vi "Happen YAML.vi"(4 "Condensed?":bool=TRUE, 6 "No Label?":bool, 8 "error in (no error)":errorcluster, 9 "Level":u32, 10 "Anything":variant, 11 "YAML String in":string) -> (0 "error out":errorcluster, 3 "YAML String out":string)   [LabVIEW 2015, in "YAML Parser.lvlib"]
uses:
  YAML Parser.lvlib
  <vilib>/Utility/Data Type/Type Definitions/Data Type.ctl
  <vilib>/Utility/Data Type/NI_Data Type.lvlib
  <vilib>/Utility/error.llb/whitespace.ctl
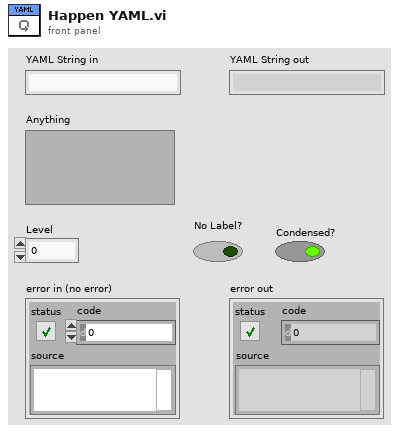
[diagram p1: front panel]
types:
  T1 = typedef "NI_Data Type.lvlib/Data Type.ctl" = enum8{"Invalid Type", "Void", "I8", "I16", "I32", "I64", "U8", "U16", "U32", "U64", "Single Float", "Double Float", "Extended Float", "Single Complex", "Double Complex", "Extended Complex", "Enum U8", "Enum U16", "Enum U32", "Enum U64", "Single Float With Unit", "Double Float With Unit", "Extended Float With Unit", "Single Complex with Unit", "Double Complex with Unit", "Extended Complex with Unit", "Boolean", "String", "Path", "Picture", "Tag", "Array", "Cluster", "Variant", "LV Variant", "Waveform", "Timestamp", "Digital Waveform", "Digital Data", "ExpressData", "Refnum", "External Data", "VI", "Poly VI", "LabVIEW Class Instance", "Fixed Point"}
  T2 = typedef "whitespace.ctl" = u16
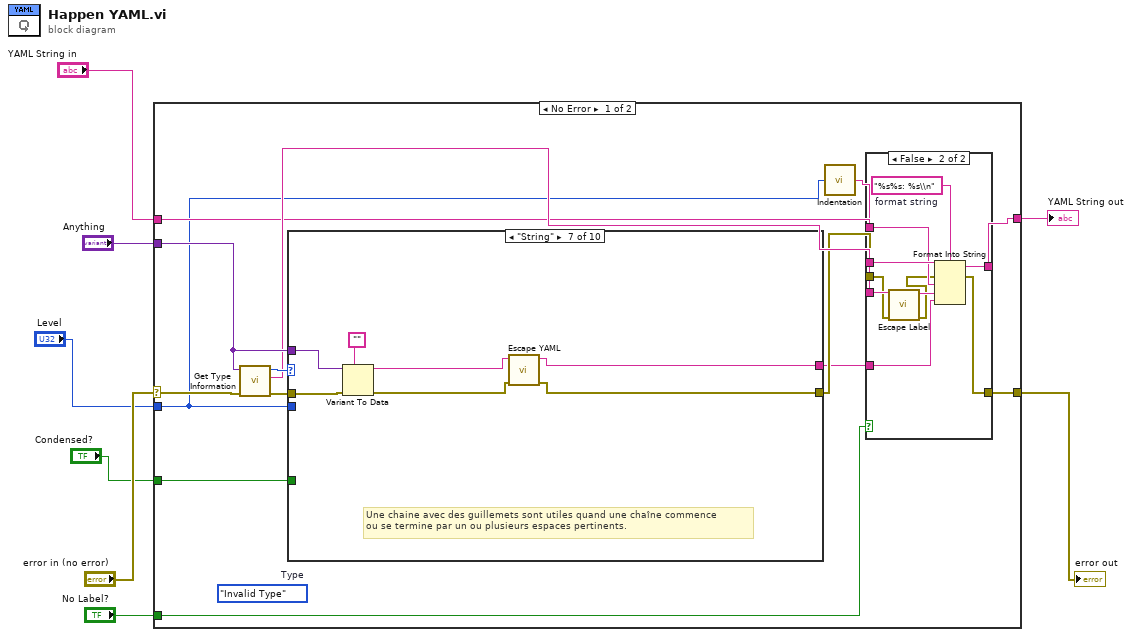
[diagram p0: block diagram]
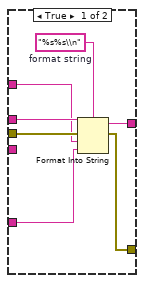
[diagram p2: hidden frame]
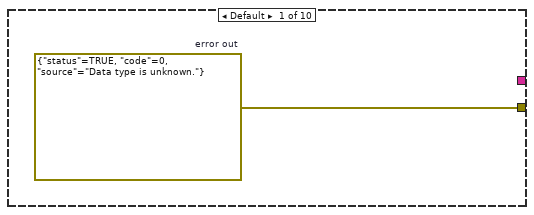
[diagram p3: hidden frame]
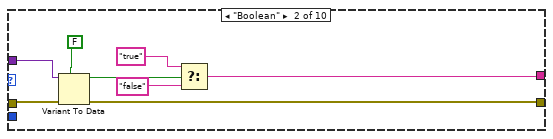
[diagram p4: hidden frame]
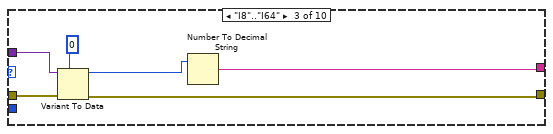
[diagram p5: hidden frame]
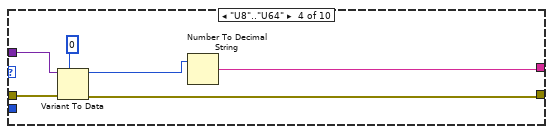
[diagram p6: hidden frame]
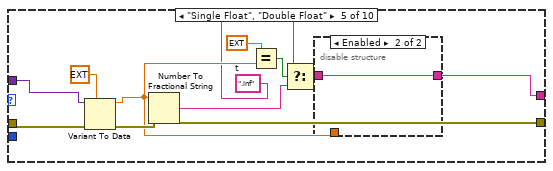
[diagram p7: hidden frame]
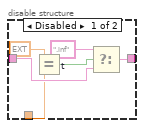
[diagram p8: hidden frame]
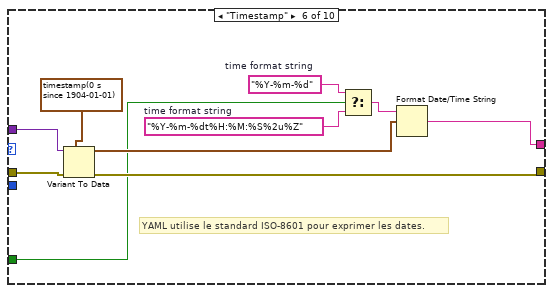
[diagram p9: hidden frame]
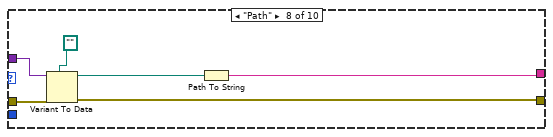
[diagram p10: hidden frame]
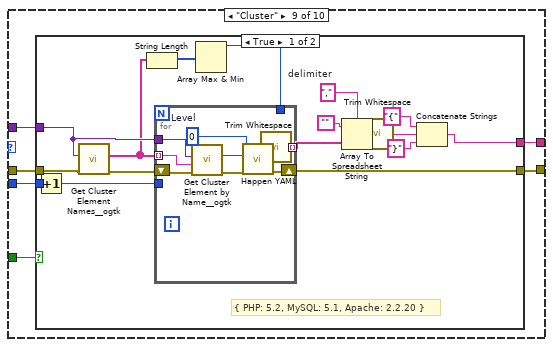
[diagram p11: hidden frame]
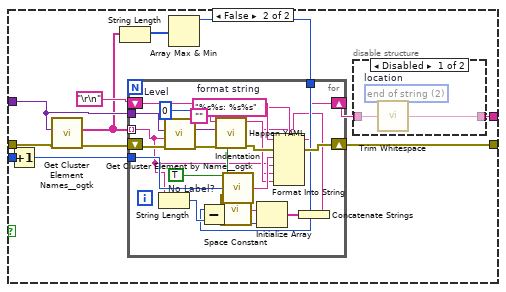
[diagram p12: hidden frame]
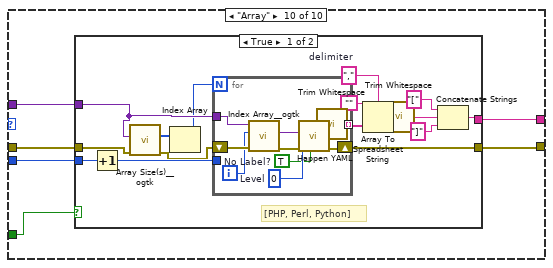
[diagram p14: hidden frame]
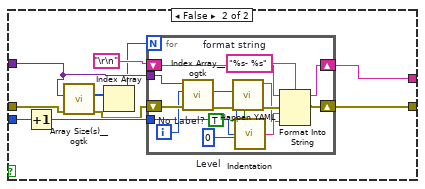
[diagram p15: hidden frame]
diagram:
  n1 = case shown="No Error" "error in (no error)" {
    selector: "error in (no error)" -> [w22 w229]
    tunnel: [w16 w229] -> w7
    tunnel: "Anything" -> [w19 _]
    tunnel: [w14 _] -> w5
    tunnel: "Level" -> [w12 _]
    tunnel: "YAML String in" -> [w13 _]
    tunnel: "No Label?" -> [w10 _]
    tunnel: "Condensed?" -> [w9 _]
    frame No Error {
      (unwired) Data_Type."Invalid Type"  # Type
      n2 = call <vilib>:"Get Type Information.vi"("error in (no error)"=w22, "Variant"=w19) -> ("error out"=w20:errorcluster, "Name"=w18:string, "Type"=w21:T1)  [unwired: 5 in, 2 out]
      n3 = case shown="\"String\"" w21 {
        tunnel: w20 -> [_ w48 w54 w60 w71 w88 w94 w101 w105 w174]
        tunnel: w19 -> [_ w47 w53 w59 w70 w87 w93 w100 w104 w173]
        tunnel: [w40 w45 w51 w57 w68 w84 w90 w96 w107 w177] -> w17
        tunnel: [_ w41 w49 w55 w61 w83 w89 w97 w103 w176] -> w15
        tunnel: w12 -> [_ _ _ _ _ _ _ _ w106 w175]
        tunnel: w9 -> [_ _ _ _ _ w82 _ _ w102 w172]
        frame Default {
          w40 = errorcluster {"status"=TRUE, "code"=0, "source"="Data type is unknown."}  # error out
        }
        frame "Boolean" {
          n4 = Variant To Data(error in=w48, type=FALSE, Variant=w47) -> (data=w44:bool, error out=w45:errorcluster)
          n5 = Select(t="true", s=w44, f="false") -> (s? t:f=w41:string)
        }
        frame "I8".."I64" {
          n6 = Variant To Data(error in=w54, type=i64 0, Variant=w53) -> (data=w50:i64, error out=w51:errorcluster)
          n7 = Number To Decimal String(number=w50) -> (decimal integer string=w49:string)  [unwired: 1 in]
        }
        frame "U8".."U64" {
          n8 = Variant To Data(error in=w60, type=u64 0, Variant=w59) -> (data=w56:u64, error out=w57:errorcluster)
          n9 = Number To Decimal String(number=w56) -> (decimal integer string=w55:string)  [unwired: 1 in]
        }
        frame "Single Float", "Double Float" {
          w62 = ".inf"  # t
          n10 = Variant To Data(error in=w71, type=ext 0.0, Variant=w70) -> (data=w63:ext, error out=w68:errorcluster)
          n11 = Number To Fractional String(number=w63) -> (F-format string=w65:string)  [unwired: 3 in]
          n12 = Equal?(x=ext inf, y=w63) -> (x = y?=w66:bool)
          n13 = Select(t=w62, s=w66, f=w65) -> (s? t:f=w64:string)
          n14 = disable-structure shown="Enabled" {
            disable-tunnel: w64 -> [w75 w78]
            disable-tunnel: w63 -> [w74 _]
            disable-tunnel: [w72 w78] -> w61
            frame Disabled {
              w73 = ".inf"  # t
              n15 = Equal?(x=ext -inf, y=w74) -> (x = y?=w76:bool)
              n16 = Select(t=w73, s=w76, f=w75) -> (s? t:f=w72:string)
            }
            frame Enabled {
            }
          }
        }
        frame "Timestamp" {
          w80 = "%Y-%m-%d"  # time format string
          w81 = "%Y-%m-%dt%H:%M:%S%2u%Z"  # time format string
          # "YAML utilise le standard ISO-8601 pour exprimer les dates."
          n17 = Variant To Data(error in=w88, type=timestamp(0 s since 1904-01-01), Variant=w87) -> (data=w85:timestamp, error out=w84:errorcluster)
          n18 = Select(t=w80, s=w82, f=w81) -> (s? t:f=w79:string)
          n19 = Format Date/Time String(time format string (%c)=w79, seconds (now)=w85) -> (date/time string=w83:string)  [unwired: 1 in]
        }
        frame "String" {
          # "Une chaine avec des guillemets sont utiles quand une chaîne commence \nou se termine par un ou plusieurs espaces pertinents."
          n20 = Variant To Data(error in=w94, type="", Variant=w93) -> (data=w92:string, error out=w91:errorcluster)
          n21 = call "Escape YAML.vi"("error in (no error)"=w91, "String"=w92) -> ("error out"=w90:errorcluster, "YAML String"=w89:string)  [unwired: 8 in]
        }
        frame "Path" {
          n22 = Variant To Data(error in=w101, type=path "", Variant=w100) -> (data=w98:path, error out=w96:errorcluster)
          n23 = Path To String(path=w98) -> (string=w97:string)
        }
        frame "Cluster" {
          n24 = case shown="True" w102 {
            tunnel: [w124 w145] -> w107
            tunnel: w106 -> [w123 w142]
            tunnel: w105 -> [w121 w140]
            tunnel: w104 -> [w119 w138]
            tunnel: [w109 w137] -> w103
            frame True {
              w115 = ","  # delimiter
              # "{ PHP: 5.2, MySQL: 5.1, Apache: 2.2.20 }"
              n25 = Increment(x=w123) -> (x+1=w122:u32)
              n26 = call <userlib>:"Get Cluster Element Names__ogtk.vi"("error in (no error)"=w121, "Cluster"=w119) -> ("error out"=w120:errorcluster, "Element Names"=w118:string[])  [unwired: 8 in]
              n27 = String Length(string=w118) -> (length=w117:i32[])
              n28 = Array Max & Min(array=w117) -> (max value=w116:i32)  [unwired: 3 out]
              n29 = for {
                shift-right: [w126] -> w124
                shift-left: w120 -> [w133]
                tunnel: w122 -> [_]
                tunnel: w118 -> [w129] mode=indexing
                tunnel: w119 -> [w132]
                tunnel: w116 -> [_]
                tunnel: [w125] -> w111 mode=indexing
                w128 = u32 0  # Level
                n30 = call <userlib>:"Get Cluster Element by Name__ogtk.vi"("error in (no error)"=w133, "Element Name"=w129, "Cluster"=w132) -> ("error out"=w131:errorcluster, "VElement"=w130:variant)  [unwired: 6 in, 1 out]
                n31 = call "Happen YAML.vi"("error in (no error)"=w131, "Level"=w128, "Anything"=w130) -> ("error out"=w126:errorcluster, "YAML String out"=w127:string)  [unwired: 7 in]
                n32 = call <vilib>:"Trim Whitespace.vi"("string"=w127) -> ("trimmed string"=w125:string)  [unwired: 1 in]
              }
              n33 = Array To Spreadsheet String(delimiter (Tab)=w115, array=w111, 3:"") -> (spreadsheet string=w114:string)
              n34 = call <vilib>:"Trim Whitespace.vi"("string"=w114) -> ("trimmed string"=w108:string)  [unwired: 1 in]
              n35 = Concatenate Strings("{", w108, "}") -> (w109:string)
            }
            frame False {
              n36 = Increment(x=w142) -> (x+1=w141:u32)
              n37 = call <userlib>:"Get Cluster Element Names__ogtk.vi"("error in (no error)"=w140, "Cluster"=w138) -> ("error out"=w139:errorcluster, "Element Names"=w136:string[])  [unwired: 8 in]
              n38 = String Length(string=w136) -> (length=w135:i32[])
              n39 = Array Max & Min(array=w135) -> (max value=w134:i32)  [unwired: 3 out]
              n40 = for {
                shift-right: [w165] -> w145
                shift-left: w139 -> [w171]
                shift-right: [w151] -> w143
                shift-left: "\r\n" -> [w164]
                tunnel: w141 -> [w162]
                tunnel: w136 -> [w158] mode=indexing
                tunnel: w138 -> [w170]
                tunnel: w134 -> [w156]
                w150 = u32 0  # Level
                w161 = "%s%s: %s%s"  # format string
                w167 = TRUE  # No Label?
                n41 = String Length(string=w158) -> (length=w157:i32)
                n42 = call <userlib>:"Get Cluster Element by Name__ogtk.vi"("error in (no error)"=w171, "Element Name"=w158, "Cluster"=w170) -> ("error out"=w169:errorcluster, "VElement"=w168:variant)  [unwired: 6 in, 1 out]
                n43 = Subtract(x=w156, y=w157) -> (x-y=w153:i32)
                n44 = call "Happen YAML.vi"("No Label?"=w167, "error in (no error)"=w169, "Level"=w150, "Anything"=w168, "YAML String in"="") -> ("error out"=w166:errorcluster, "YAML String out"=w159:string)  [unwired: 5 in]
                n45 = call <vilib>:"Space Constant.vi"() -> ("String"=w155:string)
                n46 = call "Indentation.vi"("Index"=w162) -> ("Indentation"=w160:string)
                n47 = Initialize Array(w155, w153) -> (w154:string[])
                n48 = Concatenate Strings(w154) -> (w152:string)
                n49 = Format Into String(format string=w161, initial string=w164, error in=w166, w160, w158, w152, w159) -> (resulting string=w151:string, error out=w165:errorcluster)
              }
              n50 = disable-structure shown="Disabled" {
                disable-tunnel: w143 -> [w148 w149]
                disable-tunnel: [w147 w149] -> w137
                frame Disabled {
                  w146 = T2 2 items=["both", "start of string", "end of string"]  # location
                  n51 = call <vilib>:"Trim Whitespace.vi"("string"=w148, "location (both)"=w146) -> ("trimmed string"=w147:string)
                }
                frame Enabled {
                }
              }
            }
          }
        }
        frame "Array" {
          n52 = case shown="True" w172 {
            tunnel: [w193 w213] -> w177
            tunnel: [w182 w211] -> w176
            tunnel: w175 -> [w192 w210]
            tunnel: w174 -> [w190 w208]
            tunnel: w173 -> [w189 w207]
            frame True {
              w184 = ","  # delimiter
              # "[PHP, Perl, Python]"
              n53 = Increment(x=w192) -> (x+1=w191:u32)
              n54 = call <userlib>:"Array Size(s)__ogtk.vi"("error in (no error)"=w190, "Array"=w189) -> ("error out"=w186:errorcluster, "Size(s)"=w188:u32[])  [unwired: 7 in, 1 out]
              n55 = Index Array(array=w188) -> (element=w187:u32)  [unwired: 1 in]
              n56 = for {
                N: w187 -> [_]
                shift-right: [w196] -> w193
                shift-left: w186 -> [w203]
                tunnel: w191 -> [_]
                tunnel: w189 -> [w202]
                tunnel: [w194] -> w185 mode=indexing
                i -> [w199]
                w197 = TRUE  # No Label?
                w198 = u32 0  # Level
                n57 = call <userlib>:"Index Array__ogtk.vi"("error in (no error)"=w203, "Index (1D)"=w199, "MultiD Array"=w202) -> ("error out"=w201:errorcluster, "Array Element"=w200:variant)  [unwired: 7 in]
                n58 = call "Happen YAML.vi"("No Label?"=w197, "error in (no error)"=w201, "Level"=w198, "Anything"=w200) -> ("error out"=w196:errorcluster, "YAML String out"=w195:string)  [unwired: 6 in]
                n59 = call <vilib>:"Trim Whitespace.vi"("string"=w195) -> ("trimmed string"=w194:string)  [unwired: 1 in]
              }
              n60 = Array To Spreadsheet String(delimiter (Tab)=w184, array=w185, 3:"") -> (spreadsheet string=w183:string)
              n61 = call <vilib>:"Trim Whitespace.vi"("string"=w183) -> ("trimmed string"=w178:string)  [unwired: 1 in]
              n62 = Concatenate Strings("[", w178, "]") -> (w182:string)
            }
            frame False {
              n63 = Increment(x=w210) -> (x+1=w209:u32)
              n64 = call <userlib>:"Array Size(s)__ogtk.vi"("error in (no error)"=w208, "Array"=w207) -> ("error out"=w204:errorcluster, "Size(s)"=w206:u32[])  [unwired: 7 in, 1 out]
              n65 = Index Array(array=w206) -> (element=w205:u32)  [unwired: 1 in]
              n66 = for {
                N: w205 -> [_]
                shift-right: [w222] -> w213
                shift-left: w204 -> [w228]
                shift-right: [w216] -> w211
                shift-left: "\r\n" -> [w221]
                tunnel: w209 -> [w219]
                tunnel: w207 -> [w227]
                i -> [w224]
                w214 = TRUE  # No Label?
                w215 = u32 0  # Level
                w220 = "%s- %s"  # format string
                n67 = call <userlib>:"Index Array__ogtk.vi"("error in (no error)"=w228, "Index (1D)"=w224, "MultiD Array"=w227) -> ("error out"=w226:errorcluster, "Array Element"=w225:variant)  [unwired: 7 in]
                n68 = call "Happen YAML.vi"("No Label?"=w214, "error in (no error)"=w226, "Level"=w215, "Anything"=w225) -> ("error out"=w223:errorcluster, "YAML String out"=w217:string)  [unwired: 6 in]
                n69 = call "Indentation.vi"("Index"=w219) -> ("Indentation"=w218:string)
                n70 = Format Into String(format string=w220, initial string=w221, error in=w223, w218, w217) -> (resulting string=w216:string, error out=w222:errorcluster)
              }
            }
          }
        }
      }
      n71 = call "Indentation.vi"("Index"=w12) -> ("Indentation"=w11:string)
      n72 = case shown="False" w10 {
        tunnel: w18 -> [_ w33]
        tunnel: w17 -> [w28 w31]
        tunnel: [w27 w38] -> w16
        tunnel: w15 -> [w26 w37]
        tunnel: [w25 w36] -> w14
        tunnel: w13 -> [w24 w35]
        tunnel: w11 -> [w23 w34]
        frame True {
          w29 = "%s%s\\n"  # format string
          n73 = Format Into String(format string=w29, initial string=w24, error in=w28, w23, w26) -> (resulting string=w25:string, error out=w27:errorcluster)
        }
        frame False {
          w39 = "%s%s: %s\\n"  # format string
          n74 = call "Escape Label.vi"("error in (no error)"=w31, "Label"=w33) -> ("error out"=w30:errorcluster, "YAML Label"=w32:string)  [unwired: 8 in]
          n75 = Format Into String(format string=w39, initial string=w35, error in=w30, w34, w32, w37) -> (resulting string=w36:string, error out=w38:errorcluster)
        }
      }
    }
    frame Error {
    }
  }
  "error out" <- w7
  "YAML String out" <- w5
